vi "Inverter Lados.vi"(11 "Detection Frame":T1) -> (3 "output cluster":T1)   [LabVIEW 2016]
uses:
  SSL Detection Frame.ctl
  SSL Detection Robot.ctl
  SSL Detection Ball.ctl
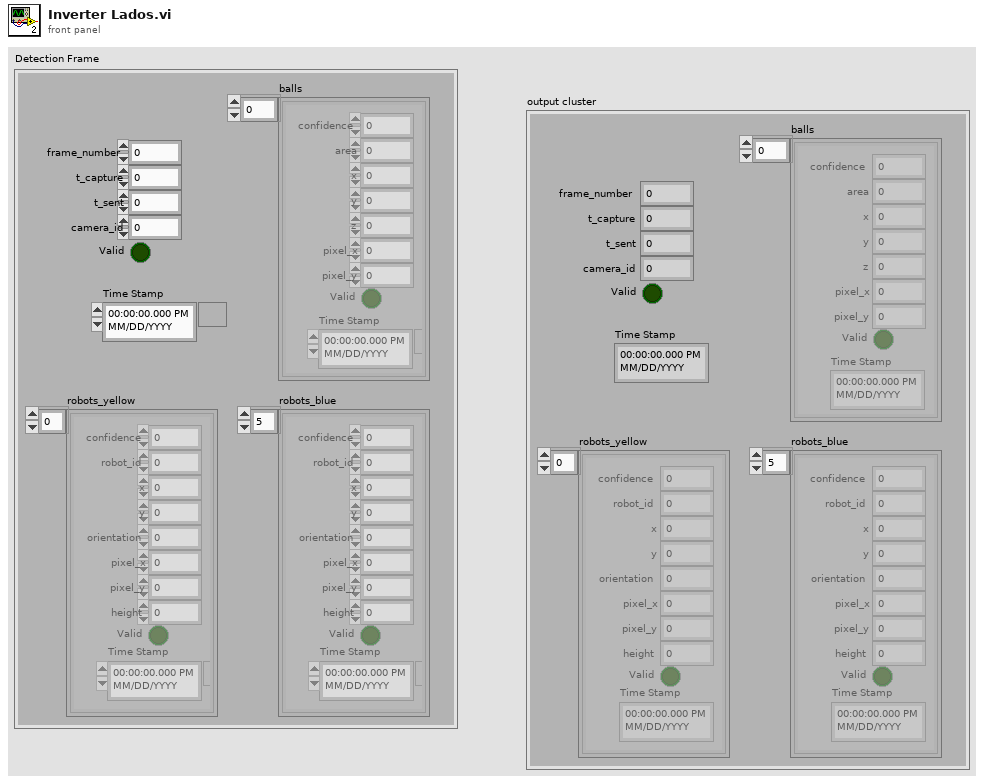
[diagram p1: front panel]
types:
  T1 = typedef "SSL Detection Frame.ctl" = cluster{"frame_number":u32, "t_capture":dbl, "t_sent":dbl, "camera_id":u32, "robots_yellow":T2[], "robots_blue":T2[], "balls":T3[], "Valid":bool, "Time Stamp":timestamp}
  T2 = typedef "SSL Detection Robot.ctl" = cluster{"x":dbl, "robot_id":u32, "confidence":sgl, "y":sgl, "orientation":sgl, "pixel_x":sgl, "pixel_y":sgl, "height":sgl, "Valid":bool, "Time Stamp":timestamp}
  T3 = typedef "SSL Detection Ball.ctl" = cluster{"x":sgl, "area":u32, "confidence":sgl, "y":sgl, "z":sgl, "pixel_x":sgl, "pixel_y":sgl, "Valid":bool, "Time Stamp":timestamp}
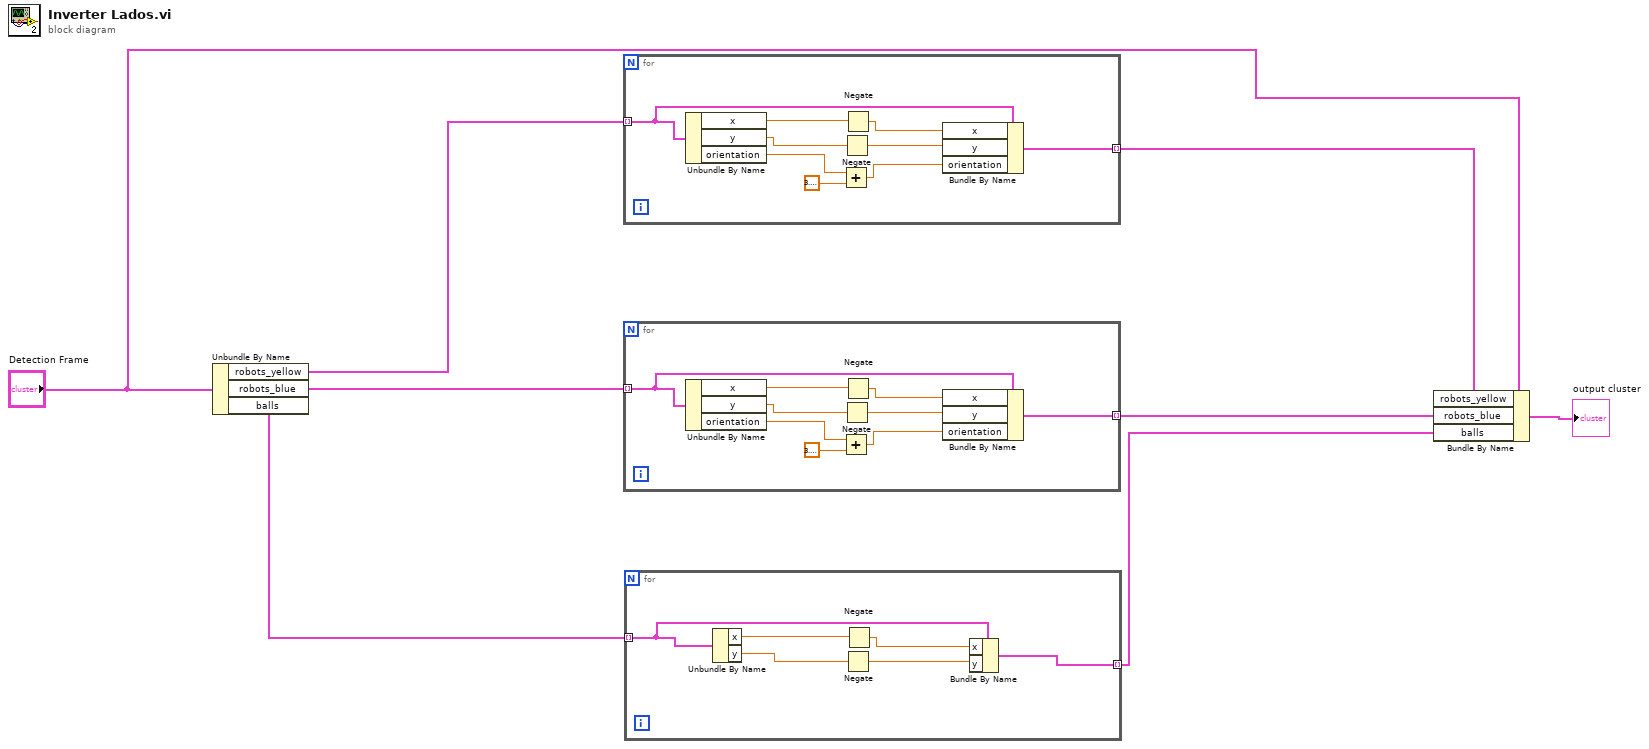
[diagram p0: block diagram]
diagram:
  n1 = Unbundle By Name("Detection Frame") -> ("robots_yellow"=w8:T2[], "robots_blue"=w6:T2[], "balls"=w4:T3[])
  n2 = for {
    tunnel: w8 -> [w13] mode=indexing
    tunnel: [w9] -> w7 mode=indexing
    n3 = Unbundle By Name(w13) -> ("x"=w17:dbl, "y"=w16:sgl, "orientation"=w14:sgl)
    n4 = Add(x=w14, y=3.141592653589793) -> (x+y=w10:dbl)
    n5 = Negate(x=w16) -> (-x=w11:sgl)
    n6 = Negate(x=w17) -> (-x=w12:dbl)
    n7 = Bundle By Name(cluster=w13, "x"=w12, "y"=w11, "orientation"=w10) -> (w9:T2)
  }
  n8 = for {
    tunnel: w6 -> [w22] mode=indexing
    tunnel: [w18] -> w5 mode=indexing
    n9 = Unbundle By Name(w22) -> ("x"=w26:dbl, "y"=w25:sgl, "orientation"=w23:sgl)
    n10 = Add(x=w23, y=3.141592653589793) -> (x+y=w19:dbl)
    n11 = Negate(x=w25) -> (-x=w20:sgl)
    n12 = Negate(x=w26) -> (-x=w21:dbl)
    n13 = Bundle By Name(cluster=w22, "x"=w21, "y"=w20, "orientation"=w19) -> (w18:T2)
  }
  n14 = for {
    tunnel: w4 -> [w30] mode=indexing
    tunnel: [w27] -> w3 mode=indexing
    n15 = Unbundle By Name(w30) -> ("x"=w32:sgl, "y"=w31:sgl)
    n16 = Negate(x=w31) -> (-x=w28:sgl)
    n17 = Negate(x=w32) -> (-x=w29:sgl)
    n18 = Bundle By Name(cluster=w30, "x"=w29, "y"=w28) -> (w27:T3)
  }
  n19 = Bundle By Name(cluster="Detection Frame", "robots_yellow"=w7, "robots_blue"=w5, "balls"=w3) -> (→"output cluster":T1)
